vi "RotateArray.vi"(1 "Method":T1(ring), 2 "Input":dbl[][](array[numeric])) -> (0 "Output":dbl[][](array[numeric]))   [LabVIEW 2012]
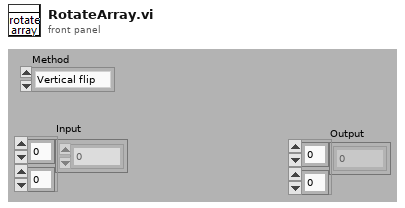
[diagram p1: front panel]
types:
  T1 = enum16{"Vertical flip", "Horizontal flip", "transpose", "rotate 90", "rotate 180", "rotate 270", "Diagonal flip"}
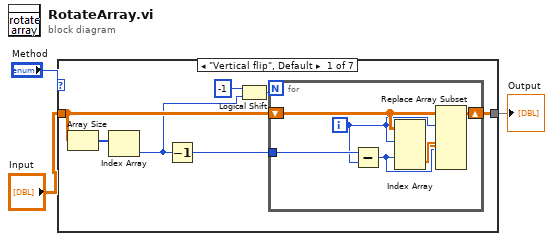
[diagram p0: block diagram]
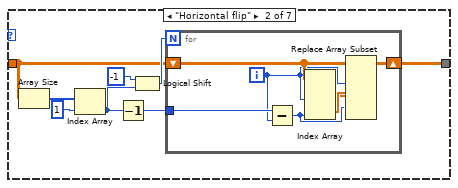
[diagram p2: hidden frame]
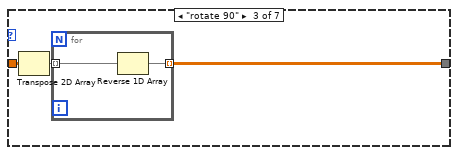
[diagram p3: hidden frame]
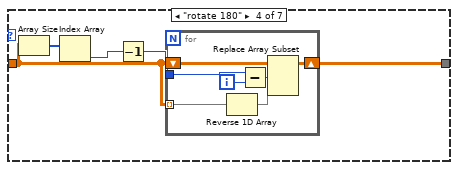
[diagram p4: hidden frame]
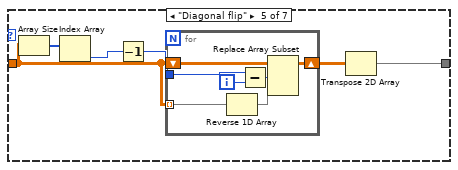
[diagram p5: hidden frame]
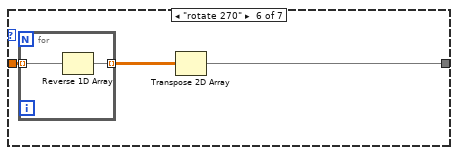
[diagram p6: hidden frame]
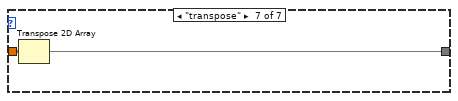
[diagram p7: hidden frame]
diagram:
  n1 = case shown="\"Vertical flip\", Default" "Method" {
    tunnel: "Input" -> [w6 w19 w34 w39 w51 w64 w69]
    tunnel: [w7 w18 w33 w38 w50 w63 w68] -> w1
    frame "Vertical flip", Default {
      n2 = Array Size(array=w6) -> (size(s)=w5:i32[])
      n3 = Index Array(array=w5) -> (element=w4:i32)  [unwired: 1 in]
      n4 = Decrement(x=w4) -> (x-1=w10:i32)
      n5 = Logical Shift(y=i8 -1, x=w4) -> (x << y=w8:i32)
      n6 = for {
        N: w8 -> [_]
        shift-right: [w17] -> w7
        shift-left: w6 -> [w16]
        tunnel: w10 -> [w13]
        i -> [w12]
        n7 = Subtract(x=w13, y=w12) -> (x-y=w11:i32)
        n8 = Index Array(array=w16, index (row) #1=w12, index (row) #2=w11) -> (element #1=w14:dbl[], element #2=w15:dbl[])  [unwired: 2 in]
        n9 = Replace Array Subset(array=w16, new element #1=w15, index (row) #1=w12, new element #2=w14, index (row) #2=w11) -> (w17:dbl[][])  [unwired: 2 in]
      }
    }
    frame "Horizontal flip" {
      n10 = Array Size(array=w19) -> (size(s)=w24:i32[])
      n11 = Index Array(array=w24, index=1) -> (element=w22:i32)
      n12 = Decrement(x=w22) -> (x-1=w20:i32)
      n13 = Logical Shift(y=i8 -1, x=w22) -> (x << y=w23:i32)
      n14 = for {
        N: w23 -> [_]
        shift-right: [w32] -> w18
        shift-left: w19 -> [w31]
        tunnel: w20 -> [w28]
        i -> [w26]
        n15 = Subtract(x=w28, y=w26) -> (x-y=w27:i32)
        n16 = Index Array(array=w31, index (col) #1=w26, index (col) #2=w27) -> (element #1=w29:dbl[], element #2=w30:dbl[])  [unwired: 2 in]
        n17 = Replace Array Subset(array=w31, new element #1=w30, index (col) #1=w26, new element #2=w29, index (col) #2=w27) -> (w32:dbl[][])  [unwired: 2 in]
      }
    }
    frame "rotate 90" {
      n18 = Transpose 2D Array(2D array=w34) -> (transposed array=w35:dbl[][])
      n19 = for {
        tunnel: w35 -> [w37] mode=indexing
        tunnel: [w36] -> w33 mode=indexing
        n20 = Reverse 1D Array(array=w37) -> (reversed array=w36:dbl[])
      }
    }
    frame "rotate 180" {
      n21 = Array Size(array=w39) -> (size(s)=w40:i32[])
      n22 = Index Array(array=w40) -> (element=w42:i32)  [unwired: 1 in]
      n23 = Decrement(x=w42) -> (x-1=w41:i32)
      n24 = for {
        shift-right: [w49] -> w38
        shift-left: w39 -> [w48]
        tunnel: w41 -> [w46]
        tunnel: w39 -> [w43] mode=indexing
        i -> [w47]
        n25 = Reverse 1D Array(array=w43) -> (reversed array=w44:dbl[])
        n26 = Subtract(x=w46, y=w47) -> (x-y=w45:i32)
        n27 = Replace Array Subset(array=w48, new element=w44, index (row)=w45) -> (w49:dbl[][])  [unwired: 1 in]
      }
    }
    frame "Diagonal flip" {
      n28 = Array Size(array=w51) -> (size(s)=w54:i32[])
      n29 = Index Array(array=w54) -> (element=w52:i32)  [unwired: 1 in]
      n30 = Decrement(x=w52) -> (x-1=w53:i32)
      n31 = for {
        shift-right: [w62] -> w55
        shift-left: w51 -> [w61]
        tunnel: w53 -> [w59]
        tunnel: w51 -> [w56] mode=indexing
        i -> [w60]
        n32 = Reverse 1D Array(array=w56) -> (reversed array=w57:dbl[])
        n33 = Subtract(x=w59, y=w60) -> (x-y=w58:i32)
        n34 = Replace Array Subset(array=w61, new element=w57, index (row)=w58) -> (w62:dbl[][])  [unwired: 1 in]
      }
      n35 = Transpose 2D Array(2D array=w55) -> (transposed array=w50:dbl[][])
    }
    frame "rotate 270" {
      n36 = for {
        tunnel: w64 -> [w67] mode=indexing
        tunnel: [w66] -> w65 mode=indexing
        n37 = Reverse 1D Array(array=w67) -> (reversed array=w66:dbl[])
      }
      n38 = Transpose 2D Array(2D array=w65) -> (transposed array=w63:dbl[][])
    }
    frame "transpose" {
      n39 = Transpose 2D Array(2D array=w69) -> (transposed array=w68:dbl[][])
    }
  }
  "Output" <- w1
